vi "configureHWIO_4_statusExpos.vi"(0 "Camera in":refnum<class "Camera.lvclass">, 1 "on":bool=TRUE, 2 "polarity":u16(ring)=1 items=["high level"=1, "low level"=2], 3 "signal_type":u32(ring)=1 items=["Status Busy", "Status Expos", "Status Line", "Status Armed"], 4 "signal_timing":u32(ring) items=["undefined", "first line", "global", "last line", "all lines"], 5 "error in (no error)":errorcluster) -> (14 "Camera out":refnum<class "Camera.lvclass">, 19 "error out":errorcluster)   [LabVIEW 2019, in "Camera.lvclass"]
doc: "Configures HWIO 4 status expose for polarity and status (enabled / disabled), and also fuction (exposure or line). Signal timing (first line, last line, all lines, global) can also be defined for the Status Expose signal. Generates an error if camera is recording or if HWIO configuration is not supported. Signal timing is ignored if the signal function is not Status Expose."
uses:
  Camera.lvclass
  pco.sdk/CameraDescription/CameraDescription.lvlib
  pco.sdk/TimingControl/TimingControl.lvlib
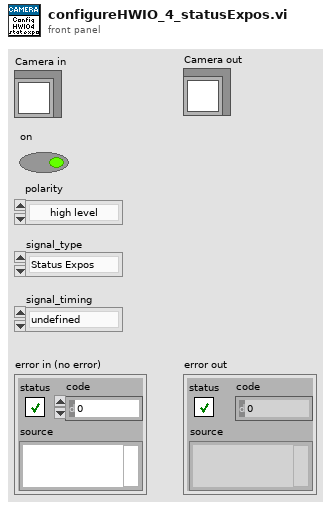
[diagram p1: front panel]
types:
  T1 = cluster{"wSensorTypeDESC":u16, "wSensorSubTypeDESC":u16, "wMaxHorzResStdDESC":u16, "wMaxVertResStdDESC":u16, "wMaxHorzResExtDESC":u16, "wMaxVertResExtDESC":u16, "wDynResDESC":u16, "wMaxBinHorzDESC":u16, "wBinHorzSteppingDESC":u16, "wMaxBinVertDESC":u16, "wBinVertSteppingDESC":u16, "wRoiHorStepsDESC":u16, "wRoiVertStepsDESC":u16, "wNumADCsDESC":u16, "wMinSizeHorzDESC":u16, "dwPixelRateDESC":u32[], "wConvFactDESC":u16[], "sCoolingSetpoints":i16[], "wSoftRoiHorStepsDESC":u16, "wSoftRoiVertStepsDESC":u16, "wIRDESC":u16, "wMinSizeVertDESC":u16, "dwMinDelayDESC":u32, "dwMaxDelayDESC":u32, "dwMinDelayStepDESC":u32, "dwMinExposureDESC":u32, "dwMaxExposureDESC":u32, "dwMinExposureStepDESC":u32, "dwMinDelayIRDESC":u32, "dwMaxDelayIRDESC":u32, "dwMinExposureIRDESC":u32, "dwMaxExposureIRDESC":u32, "wTimeTableDESC":u16, "wDoubleImageDESC":u16, "sMinCoolSetDESC":i16, "sMaxCoolSetDESC":i16, "sDefaultCoolSetDESC":i16, "wPowerDownModeDESC":u16, "wOffsetRegulationDESC":u16, "wColorPatternDESC":u16, "wPatternTypeDESC":u16, "wNumCoolingSetpoints":u16, "dwGeneralCapsDESC1":u32, "dwGeneralCapsDESC2":u32, "dwExtSyncFrequency":u32[], "dwGeneralCapsDESC3":u32, "dwGeneralCapsDESC4":u32}
  T2 = cluster{"wSignalNum":u16, "wEnabled":u16, "wType":u16, "wPolarity":u16, "wFilterSetting":u16, "wSelected":u16, "dwParameter":u32[], "dwSignalFunctionality":u32[]}
  T3 = cluster{"strSignalName":string[], "wSignalDefinitions":u16, "wSignalTypes":u16, "wSignalPolarity":u16, "wSignalFilter":u16}
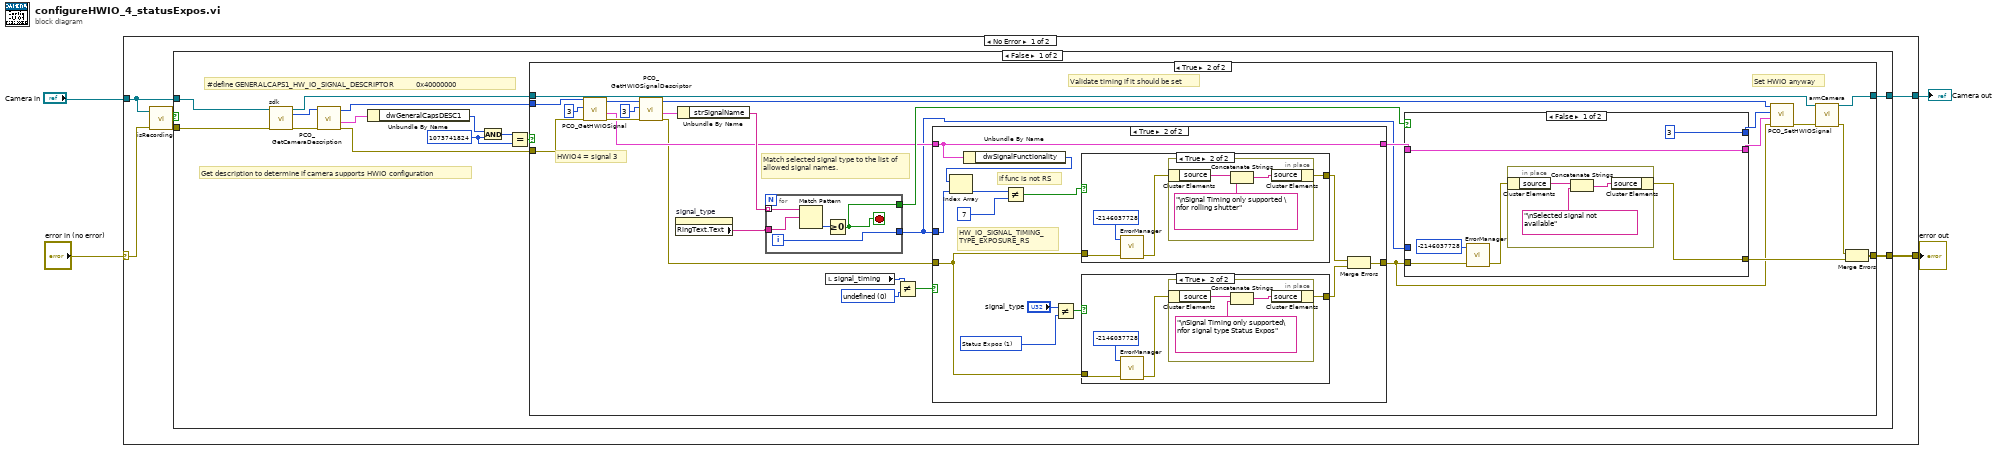
[diagram p0: block diagram]
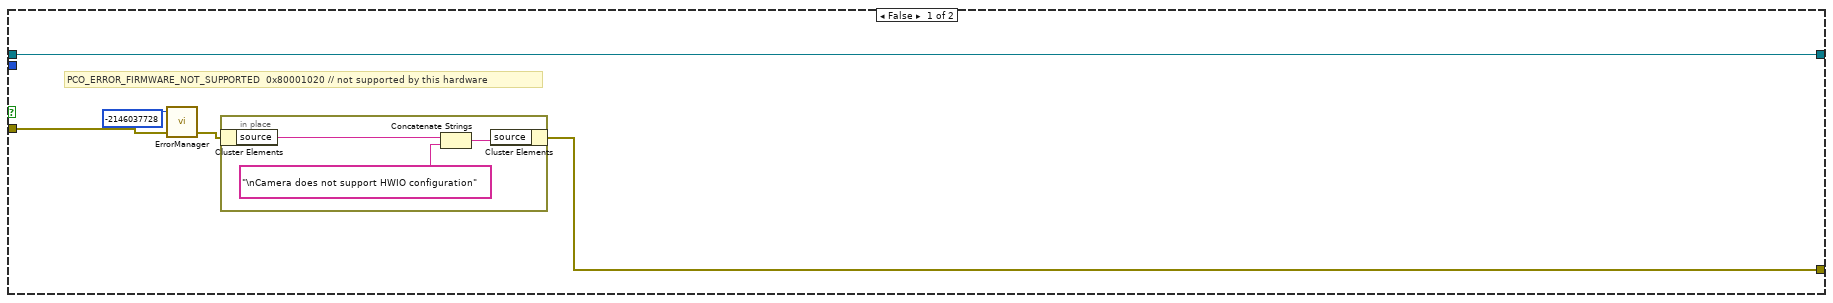
[diagram p2: hidden frame]
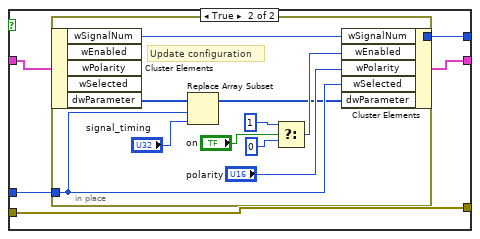
[diagram p6: hidden frame]
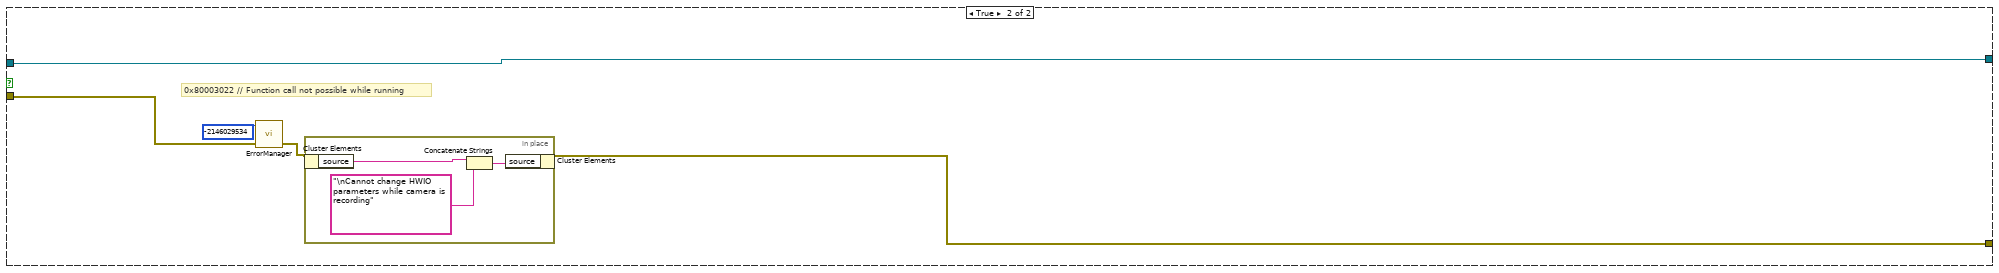
[diagram p7: hidden frame]
diagram:
  n1 = case shown="No Error" "error in (no error)" {
    selector: "error in (no error)" -> [w6 w129]
    tunnel: [w8 w129] -> w3
    tunnel: "Camera in" -> [w10 w128]
    tunnel: [w7 w128] -> w1
    frame No Error {
      n2 = call-dynamic "isRecording.vi"("Camera in"=w10, "error in (no error)"=w6) -> ("recording"=w9:bool, "error out"=w5:errorcluster)  [unwired: 11 in, 1 out]
      n3 = case shown="False" w9 {
        tunnel: w10 -> [w24 w120]
        tunnel: w5 -> [w12 w123]
        tunnel: [w15 w121] -> w8
        tunnel: [w14 w120] -> w7
        frame False {
          w19 = u32 1073741824 ("y")
          # "Get description to determine if camera supports HWIO configuration"
          # "#define GENERALCAPS1_HW_IO_SIGNAL_DESCRIPTOR           0x40000000"
          n4 = call-dynamic "sdk.vi"("Camera in"=w24, "error in (no error)"=w12) -> ("Camera out"=w16:refnum<class "Camera.lvclass">, "sdk"=w23:u64, "error out"=w13:errorcluster)  [unwired: 11 in]
          n5 = call "PCO_GetCameraDescription.vi"("error in (no error)"=w13, "ph"=w23) -> ("error out"=w11:errorcluster, "strDescription"=w22:T1, "ph out"=w17:u64)  [unwired: 6 in, 1 out]
          n6 = Unbundle By Name(w22) -> ("dwGeneralCapsDESC1"=w21:u32)
          n7 = And(x=w21, y=w19) -> (x .and. y?=w20:u32)
          n8 = Equal?(x=w20, y=w19) -> (x = y?=w18:bool)
          n9 = case shown="True" w18 {
            tunnel: w11 -> [w29 w58]
            tunnel: [w26 w45] -> w15
            tunnel: w17 -> [_ w59]
            tunnel: w16 -> [w25 w34]
            tunnel: [w25 w33] -> w14
            frame False {
              # "PCO_ERROR_FIRMWARE_NOT_SUPPORTED  0x80001020 // not supported by this hardware"
              n10 = call "ErrorManager.vi"("error in (no error)"=w29, "error code"=-2146037728) -> ("error out"=w27:errorcluster)  [unwired: 2 in, 1 out]
              n11 = in-place {
                n12 = in-place-cluster #1(w27) -> ("source"=w32:string)
                n13 = Concatenate Strings(w32, "\nCamera does not support HWIO configuration") -> (w30:string)
                n14 = in-place-cluster #1("source"=w30) -> (w26:errorcluster)
              }
            }
            frame True {
              w41 = u16 0 items=["undefined", "first line", "global", "last line", "all lines"] ("signal_timing")
              # "Validate timing if it should be set"
              # "Set HWIO anyway"
              # "Match selected signal type to the list of allowed signal names."
              # "HWIO4 = signal 3"
              n15 = call "PCO_GetHWIOSignal.vi"("error in (no error)"=w58, "wSignalNum"=u16 3, "ph"=w59) -> ("error out"=w53:errorcluster, "strSignal"=w40:T2, "ph out"=w52:u64)  [unwired: 5 in, 1 out]
              n16 = call "PCO_GetHWIOSignalDescriptor.vi"("error in (no error)"=w53, "wSignalNum"=u16 3, "ph"=w52) -> ("error out"=w37:errorcluster, "strSignalDesc"=w49:T3, "ph out"=w51:u64)  [unwired: 5 in, 1 out]
              n17 = property on="signal_type" class="Ring (strict)"() -> ("RingText.Text"=w46:string)  [unwired: 2 in, 2 out]
              n18 = Unbundle By Name(w49) -> ("strSignalName"=w48:string[])
              n19 = for {
                tunnel: w48 -> [w119] mode=indexing
                tunnel: [w116] -> w35
                tunnel: [w115] -> w47
                tunnel: w46 -> [w117]
                i -> [w116]
                stop <- w115 stop-if-true
                n20 = Match Pattern(string=w119, regular expression=w117) -> (offset past match=w118:i32)  [unwired: 1 in, 3 out]
                n21 = Greater Or Equal To 0?(x=w118) -> (x >= 0?=w115:bool)
              }
              n22 = local read "signal_timing"() -> (w42:u32)
              n23 = Not Equal?(x=w42, y=w41) -> (x != y?=w38:bool)
              n24 = case shown="True" w38 {
                tunnel: w40 -> [w61 w74]
                tunnel: [w61 w74] -> w39
                tunnel: w37 -> [w60 w66]
                tunnel: [w60 w65] -> w36
                tunnel: w35 -> [_ w73]
                frame False {
                }
                frame True {
                  w62 = u32 1 items=["Status Busy", "Status Expos", "Status Line", "Status Armed"] ("signal_type")
                  # "HW_IO_SIGNAL_TIMING_\nTYPE_EXPOSURE_RS"
                  # "if func is not RS"
                  n25 = Unbundle By Name(w74) -> ("dwSignalFunctionality"=w72:u32[])
                  n26 = Index Array(array=w72, index=w73) -> (element=w71:u32)
                  n27 = Not Equal?(x=w71, y=u32 7) -> (x != y?=w68:bool)
                  n28 = Not Equal?(x="signal_type", y=w62) -> (x != y?=w67:bool)
                  n29 = case shown="True" w68 {
                    tunnel: w66 -> [w83 w85]
                    tunnel: [w83 w84] -> w64
                    frame False {
                    }
                    frame True {
                      n30 = call "ErrorManager.vi"("error in (no error)"=w85, "error code"=-2146037728) -> ("error out"=w86:errorcluster)  [unwired: 2 in, 1 out]
                      n31 = in-place {
                        n32 = in-place-cluster #2(w86) -> ("source"=w90:string)
                        n33 = Concatenate Strings(w90, "\nSignal Timing only supported \nfor rolling shutter" ("string")) -> (w89:string)
                        n34 = in-place-cluster #2("source"=w89) -> (w84:errorcluster)
                      }
                    }
                  }
                  n35 = case shown="True" w67 {
                    tunnel: w66 -> [w75 w77]
                    tunnel: [w75 w76] -> w63
                    frame False {
                    }
                    frame True {
                      n36 = call "ErrorManager.vi"("error in (no error)"=w77, "error code"=-2146037728) -> ("error out"=w78:errorcluster)  [unwired: 2 in, 1 out]
                      n37 = in-place {
                        n38 = in-place-cluster #3(w78) -> ("source"=w82:string)
                        n39 = Concatenate Strings(w82, "\nSignal Timing only supported\nfor signal type Status Expos" ("string")) -> (w81:string)
                        n40 = in-place-cluster #3("source"=w81) -> (w76:errorcluster)
                      }
                    }
                  }
                  n41 = Merge Errors(w64, w63) -> (w65:errorcluster)
                }
              }
              n42 = case shown="False" w47 {
                tunnel: w39 -> [w96 w104]
                tunnel: [u16 3 ("wSignalNum") w103] -> w56
                tunnel: [w96 w102] -> w55
                tunnel: w36 -> [w94 w101]
                tunnel: [w91 w101] -> w43
                tunnel: w35 -> [_ w100]
                frame False {
                  n43 = call "ErrorManager.vi"("error in (no error)"=w94, "error code"=-2146037728) -> ("error out"=w92:errorcluster)  [unwired: 2 in, 1 out]
                  n44 = in-place {
                    n45 = in-place-cluster #4(w92) -> ("source"=w99:string)
                    n46 = Concatenate Strings(w99, "\nSelected signal not available" ("string")) -> (w98:string)
                    n47 = in-place-cluster #4("source"=w98) -> (w91:errorcluster)
                  }
                }
                frame True {
                  n48 = in-place {
                    in-place-border: [w109] -> w103
                    in-place-border: w100 -> [w107]
                    # "Update configuration"
                    n49 = in-place-cluster #5(w104) -> ("wSignalNum"=w109:u16, "dwParameter"=w108:u32[])  [unwired: 3 out]
                    n50 = Replace Array Subset(array=w108, new element="signal_timing", index=w107) -> (w105:u32[])
                    n51 = Select(t=u16 1 ("wEnabled"), s="on", f=u16 0 ("wEnabled")) -> (s? t:f=w112:u16)
                    n52 = in-place-cluster #5("wSignalNum"=w109, "wEnabled"=w112, "wPolarity"="polarity", "wSelected"=w107, "dwParameter"=w105) -> (w102:T2)
                  }
                }
              }
              n53 = call "PCO_SetHWIOSignal.vi"("error in (no error)"=w36, "strSignal"=w55, "wSignalNum"=w56, "ph"=w51) -> ("error out"=w54:errorcluster)  [unwired: 5 in, 2 out]
              n54 = call-dynamic "armCamera.vi"("Camera in"=w34, "error in (no error)"=w54) -> ("Camera out"=w33:refnum<class "Camera.lvclass">, "error out"=w44:errorcluster)  [unwired: 12 in]
              n55 = Merge Errors(w44, w43) -> (w45:errorcluster)
            }
          }
        }
        frame True {
          # "0x80003022 // Function call not possible while running"
          n56 = call "ErrorManager.vi"("error in (no error)"=w123, "error code"=-2146029534) -> ("error out"=w122:errorcluster)  [unwired: 2 in, 1 out]
          n57 = in-place {
            n58 = in-place-cluster #6(w122) -> ("source"=w127:string)
            n59 = Concatenate Strings(w127, "\nCannot change HWIO parameters while camera is recording") -> (w125:string)
            n60 = in-place-cluster #6("source"=w125) -> (w121:errorcluster)
          }
        }
      }
    }
    frame Error {
    }
  }
  "Camera out" <- w1
  "error out" <- w3
